vi "HAPS_PhaseGainSweep_Preamp_ICs.vi"() -> ()   [LabVIEW 2023, in "HAPS.lvlib"]
uses:
  HAPS.lvlib
  HAPS_SerialPort.ctl
  MCU_Function.ctl
  set_ele.ctl
  HAPS_MCU_ELE_Func.ctl
  R_S/R_S.lvlib
panel:
  out "Each_Phase_Sweep(sec)":dbl
  out "dup path":path
  out "Gain_step":i32
  out "channel":i32
  out "chain_id":i32
  out "group":i32
  out "array_id":i32
  in  "Gain_Start_Step":i32
  in  "Phase Sweep Step":i32=64
  in  "Gain Sweep Step":i32=36
  in  "comn_gain":i32=17
  in  "Init?":bool=TRUE
  in  "File_note":string
  out "Duration(sec)":dbl
  out "In-Phase : Phase(degree)":dbl[](graph)
  out "In-Phase : Gain(dB)":dbl[](graph)
  in  "Phase diff. Criteria":dbl format="%#_13g"
  in  "Tx/Rx":enum16{"Rx", "Tx"}(ring)=enum."Tx"
  in  "array_id (MCU index)":i32
  in  "MCU_UART_addr":refnum<visa-resource-name>="COM8"
  in  "Target(degree)":dbl format="%#_13g"
  in  "SweepPoints":i32=11
  in  "sParameter":i32=21
  in  "Stop_Freq(GHz)":dbl=39.5
  in  "Start_Freq(GHz)":dbl=38.5
  in  "VISA resource name":refnum<visa-resource-name>="TCPIP0::192.168.119.45::inst0::INSTR"
  in  "HAPS_Equipment":enum16{"Keysight", "R&S"}(ring)=enum."R&S"
  # "HAPS_24x24_PhaseGain_Sweep_Preamp_v1.4"
  # "K:4718\nR:2798"
  # "VNA"
  # "Test Status"
  # "DUT"
  # "TCPIP0::192.168.1.31::hislip0::INSTR"
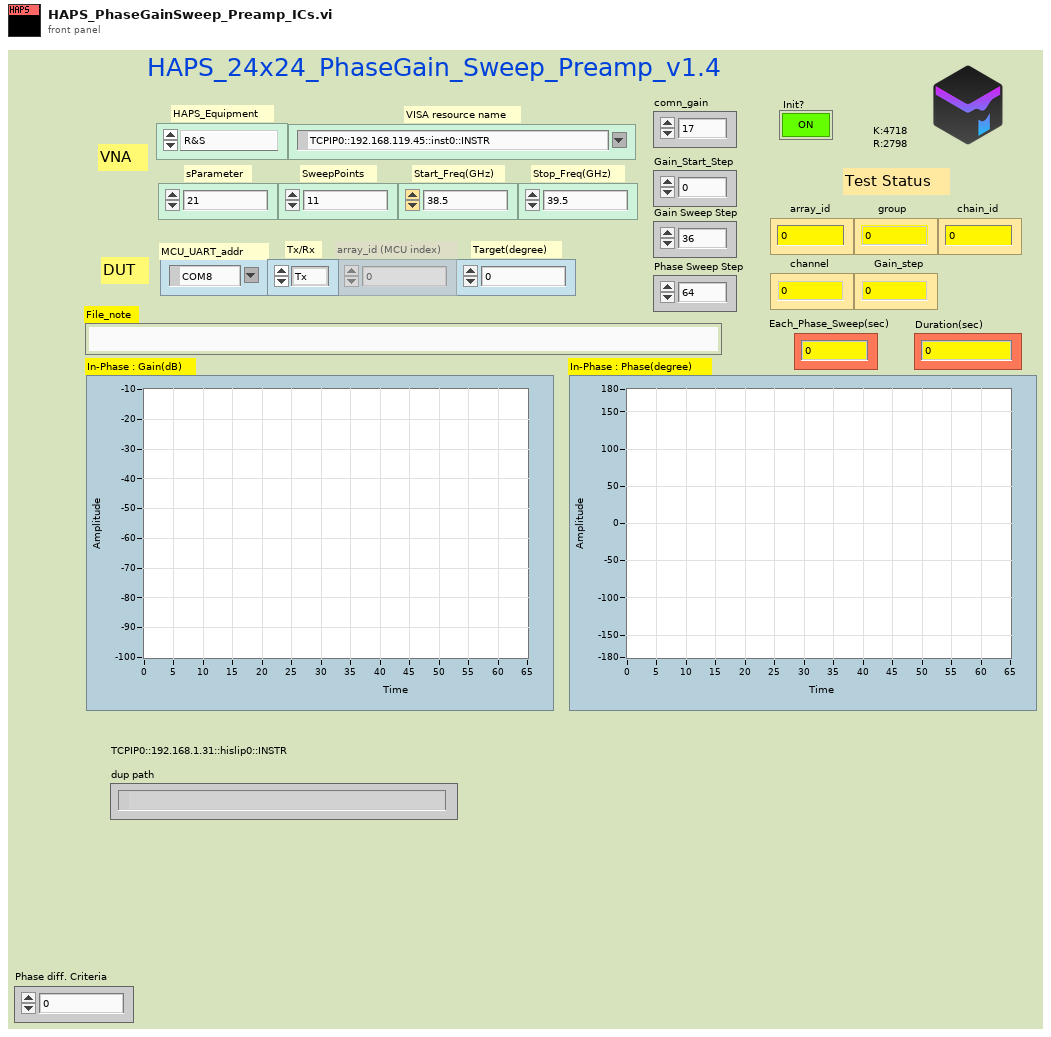
[diagram p1: front panel]
types:
  T1 = typedef "HAPS.lvlib/HAPS_SerialPort.ctl" = enum16{"Init", "Close", "CMD", "Flush"}
  T2 = typedef "HAPS.lvlib/HAPS_MCU_ELE_Func.ctl" = enum16{"array_init", "set_com_gain", "set_ch_gain_phase", "set_pd_range", "get_preamp_temp", "get_bfic_temp", "get_tx_pd", "ch_on", "ch_on_2", "ch_ctrl_all", "array_ctrl_src"}
  T3 = typedef "HAPS.lvlib/MCU_Function.ctl" = cluster{"Tx/Rx":enum16{"Rx", "Tx"}, "Enable?":enum16{"OFF", "On"}, "Source":enum16{"MCU", "ACU"}}
  T4 = typedef "HAPS.lvlib/set_ele.ctl" = cluster{"ch":i32, "chain_id":i32, "group":i32, "array_id":i32, "ele_phase":i32, "ele_gain":i32, "com_gain":i32, "pd_range":i32}
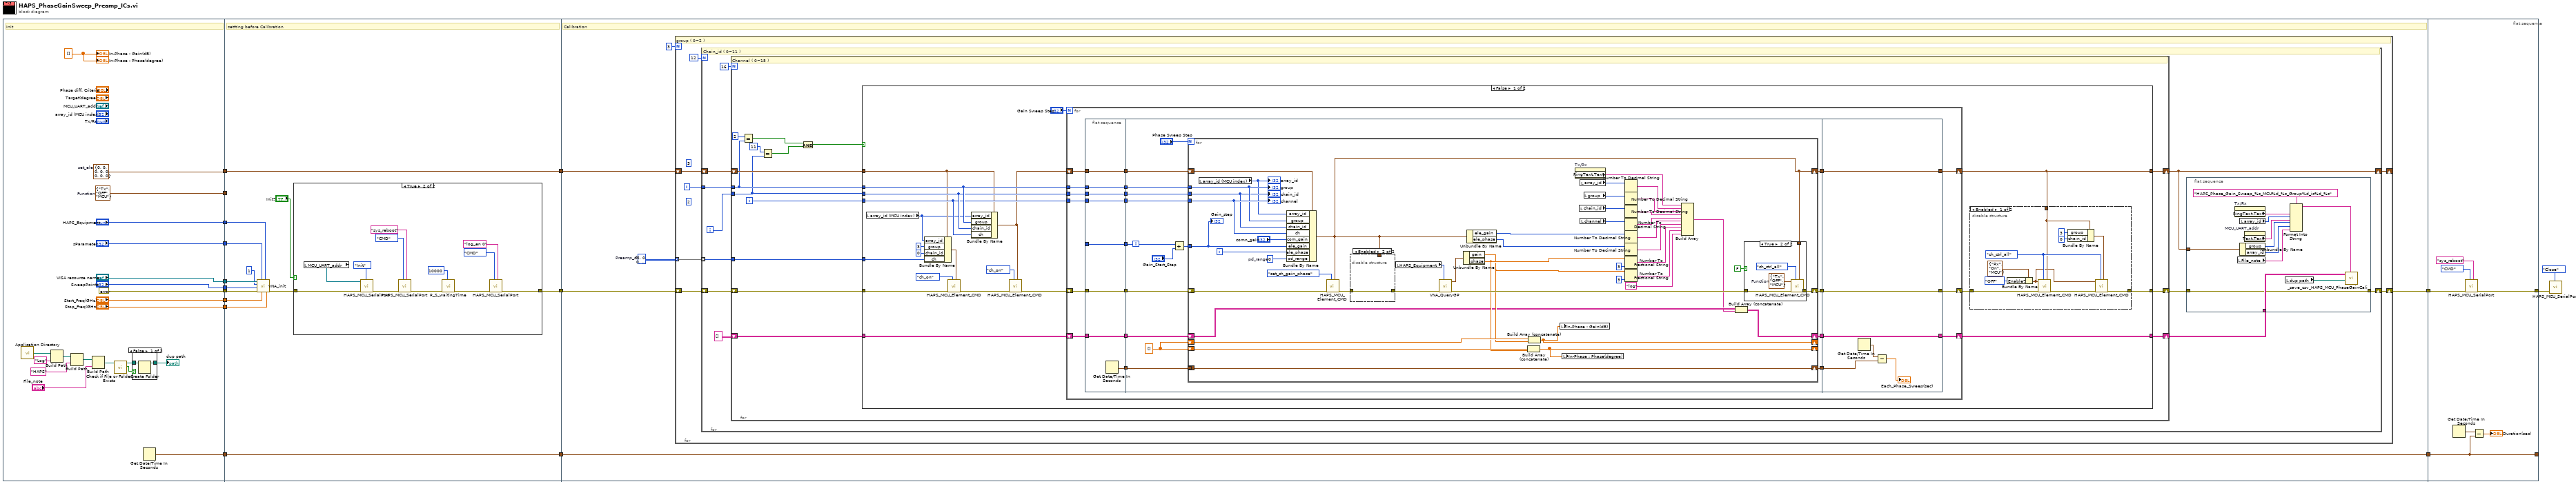
[diagram p0: block diagram]
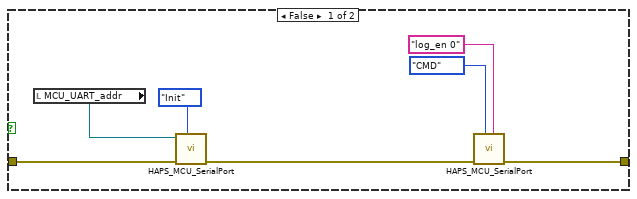
[diagram p3: hidden frame]
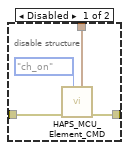
[diagram p4: hidden frame]
diagram:
  n1 = flat-sequence {
    tunnel: [w31] -> w17
    tunnel: [w38] -> w16
    tunnel: [errorcluster {"status"=FALSE, "code"=0, "source"=""} ("error in")] -> w14
    tunnel: ["sParameter"] -> w12
    tunnel: ["VISA resource name"] -> w11
    tunnel: ["Start_Freq(GHz)"] -> w10
    tunnel: ["Stop_Freq(GHz)"] -> w9
    tunnel: ["SweepPoints"] -> w8
    tunnel: ["HAPS_Equipment"] -> w7
    tunnel: [w28] -> w5
    tunnel: w17 -> [w54]
    tunnel: w16 -> [_]
    tunnel: [w54] -> w15
    tunnel: w14 -> [w53]
    tunnel: [w45] -> w13
    tunnel: w12 -> [w52]
    tunnel: w11 -> [w51]
    tunnel: w10 -> [w50]
    tunnel: w9 -> [w49]
    tunnel: w8 -> [w48]
    tunnel: w7 -> [w44]
    tunnel: [w43] -> w6
    tunnel: w5 -> [w43]
    tunnel: w15 -> [w78]
    tunnel: w13 -> [w79]
    tunnel: w6 -> [w76]
    tunnel: [w76] -> w4
    tunnel: [w74] -> w3
    tunnel: [w276] -> _
    tunnel: w4 -> [w276]
    tunnel: w3 -> [w272]
    tunnel: [w271] -> w2
    frame #0 {
      w29 = dbl[] []
      w31 = T4 {"ch"=0, "chain_id"=0, "group"=0, "array_id"=0, "ele_phase"=0, "ele_gain"=0, "com_gain"=0, "pd_range"=0}  # set_ele
      w38 = T3 {"Tx/Rx"=enum."Tx", "Enable?"=enum."OFF", "Source"=enum."MCU"}  # Function
      # "Init"
      n2 = call <vilib>:"Application Directory.vi"() -> ("Application Directory"=w26:path)
      n3 = Build Path(base path=w26, name or relative path="Log") -> (appended path=w27:path)
      n4 = Build Path(base path=w27, name or relative path="HAPS") -> (appended path=w23:path)
      n5 = Build Path(base path=w23, name or relative path="File_note") -> (appended path=w21:path)
      n6 = call <vilib>:"Check if File or Folder Exists.vi"("path"=w21) -> ("file or folder exists?"=w20:bool, "dup path"=w19:path)  [unwired: 8 in, 1 out]
      n7 = case shown="False" w20 {
        tunnel: w19 -> [w40 w41]
        tunnel: [w39 w41] -> w18
        frame False {
          n8 = Create Folder(path (use dialog)=w40) -> (created path=w39:path)  [unwired: 2 in, 2 out]
        }
        frame True {
        }
      }
      "dup path" <- w18
      n9 = Get Date/Time In Seconds() -> (seconds since 1Jan1904=w28:timestamp)
      "In-Phase : Gain(dB)" <- w29
      "In-Phase : Phase(degree)" <- w29
    }
    frame #1 {
      # "settting before Calibration"
      n10 = call "VNA_init.vi"("Stop_Freq(GHz)"=w49, "HAPS_MCU_CMD"=w44, "Start_Freq(GHz)"=w50, "sParameter"=w52, "error in"=w53, "SweepPoints"=w48, "Mark no."=1, "VISA resource name"=w51) -> ("error out"=w46:errorcluster)  [unwired: 3 in]
      n11 = case shown="True" "Init?" {
        tunnel: w46 -> [w58 w71]
        tunnel: [w55 w68] -> w45
        frame False {
          n12 = local read "MCU_UART_addr"() -> (w56:refnum<visa-resource-name>)
          n13 = call "HAPS_MCU_SerialPort.vi"("HAPS_SerialPort_Func"=HAPS_SerialPort."Init", "error in"=w58, "VISA resource name"=w56) -> ("error out"=w59:errorcluster)  [unwired: 6 in, 2 out]
          n14 = call "HAPS_MCU_SerialPort.vi"("Command"="log_en 0", "HAPS_SerialPort_Func"=enum16{"Init", "Close", "CMD"}."CMD" ("HAPS_SerialPort"), "error in"=w59) -> ("error out"=w55:errorcluster)  [unwired: 6 in, 2 out]
        }
        frame True {
          n15 = local read "MCU_UART_addr"() -> (w69:refnum<visa-resource-name>)
          n16 = call "HAPS_MCU_SerialPort.vi"("HAPS_SerialPort_Func"=HAPS_SerialPort."Init", "error in"=w71, "VISA resource name"=w69) -> ("error out"=w65:errorcluster)  [unwired: 6 in, 2 out]
          n17 = call "HAPS_MCU_SerialPort.vi"("Command"="sys_reboot", "HAPS_SerialPort_Func"=enum16{"Init", "Close", "CMD"}."CMD" ("HAPS_SerialPort"), "error in"=w65) -> ("error out"=w64:errorcluster)  [unwired: 6 in, 2 out]
          n18 = call "R_S_waitingTime.vi"("Waiting Time(ms)"=u32 10000, "error in"=w64) -> ("error out"=w63:errorcluster)  [unwired: 9 in]
          n19 = call "HAPS_MCU_SerialPort.vi"("Command"="log_en 0", "HAPS_SerialPort_Func"=enum16{"Init", "Close", "CMD"}."CMD" ("HAPS_SerialPort"), "error in"=w63) -> ("error out"=w68:errorcluster)  [unwired: 6 in, 2 out]
        }
      }
    }
    frame #2 {
      w75 = i32[][] [[2, 0, 0, 8, 8, 10, 11, 9, 9, 1, 1, 3], [3, 1, 1, 9, 9, 11, 13, 15, 15, 7, 7, 5], [5, 7, 7, 15, 15, 13, 14, 14, 6, 6, 4, 12]]  # Preamp_ch
      # "Calibration"
      n20 = for {
        N: 3 -> [_]
        shift-right: [w80] -> _
        shift-left: w78 -> [w84]
        shift-right: [w86] -> w74
        shift-left: w79 -> [w85]
        tunnel: w75 -> [w81] mode=indexing
        i -> [w82]
        (unwired) 2
        (unwired) 3
        # "group ( 0~2 )"
        n21 = for {
          N: 12 -> [_]
          shift-right: [w91] -> w80
          shift-left: w84 -> [w95]
          shift-right: [w87] -> w86
          shift-left: w85 -> [w96]
          tunnel: w82 -> [w94]
          tunnel: w81 -> [w92] mode=indexing
          i -> [w93]
          # "Chain_id ( 0~11 )"
          n22 = for {
            N: 16 -> [_]
            shift-right: [w121] -> w91
            shift-left: w95 -> [w124]
            shift-right: [w119] -> w90
            shift-left: string[][] [] -> [w120]
            shift-right: [w122] -> w88
            shift-left: w96 -> [w123]
            tunnel: w94 -> [w118]
            tunnel: w93 -> [w111]
            tunnel: w92 -> [w110]
            i -> [w112]
            # "Channel ( 0~15 )"
            n23 = Equal?(x=2, y=w118) -> (x = y?=w115:bool)
            n24 = Equal?(x=11, y=w111) -> (x = y?=w114:bool)
            n25 = And(x=w115, y=w114) -> (x .and. y?=w113:bool)
            n26 = case shown="False" w113 {
              tunnel: w124 -> [w133 w269]
              tunnel: w112 -> [w142 _]
              tunnel: w123 -> [w134 w268]
              tunnel: w118 -> [w144 _]
              tunnel: w111 -> [w143 _]
              tunnel: [w138 w268] -> w122
              tunnel: [w137 w269] -> w121
              tunnel: w120 -> [w145 w270]
              tunnel: [w126 w270] -> w119
              tunnel: w110 -> [w128 _]
              frame False {
                n27 = local read "array_id (MCU index)"() -> (w131:i32)
                n28 = Bundle By Name(cluster=w133, "array_id"=w131, "group"=3, "chain_id"=0, "ch"=w128) -> (w132:T4)
                n29 = call "HAPS_MCU_Element_CMD.vi"("set_ele"=w132, "HAPS_MCU_ELE_Func."=HAPS_MCU_ELE_Func."ch_on", "error in"=w134) -> ("error out"=w135:errorcluster)  [unwired: 7 in, 1 out]
                n30 = Bundle By Name(cluster=w133, "array_id"=w131, "group"=w144, "chain_id"=w143, "ch"=w142) -> (w127:T4)
                n31 = call "HAPS_MCU_Element_CMD.vi"("set_ele"=w127, "HAPS_MCU_ELE_Func."=HAPS_MCU_ELE_Func."ch_on", "error in"=w135) -> ("error out"=w140:errorcluster)  [unwired: 7 in, 1 out]
                n32 = for {
                  N: "Gain Sweep Step" -> [_]
                  tunnel: w144 -> [w166]
                  tunnel: w143 -> [w165]
                  tunnel: w142 -> [w164]
                  shift-right: [w162] -> w139
                  shift-left: w140 -> [w163]
                  shift-right: [w161] -> w137
                  shift-left: w127 -> [w160]
                  shift-right: [w159] -> w126
                  shift-left: w145 -> [w167]
                  i -> [w158]
                  n33 = flat-sequence {
                    tunnel: w158 -> [w169]
                    tunnel: w160 -> [w170]
                    tunnel: w163 -> [w171]
                    tunnel: w164 -> [w172]
                    tunnel: w165 -> [w173]
                    tunnel: w166 -> [w174]
                    tunnel: w167 -> [w175]
                    tunnel: [w175] -> w157
                    tunnel: [w174] -> w156
                    tunnel: [w173] -> w155
                    tunnel: [w172] -> w154
                    tunnel: [w171] -> w153
                    tunnel: [w170] -> w152
                    tunnel: [w169] -> w151
                    tunnel: [w168] -> w150
                    tunnel: w157 -> [w190]
                    tunnel: w156 -> [w189]
                    tunnel: w155 -> [w188]
                    tunnel: w154 -> [w187]
                    tunnel: w153 -> [w186]
                    tunnel: w152 -> [w183]
                    tunnel: w151 -> [w181]
                    tunnel: w150 -> [w177]
                    tunnel: [w185] -> w149
                    tunnel: [w184] -> w148
                    tunnel: [w182] -> w147
                    tunnel: [w176] -> w146
                    tunnel: [w253] -> w159
                    tunnel: [w254] -> w161
                    tunnel: [w255] -> w162
                    tunnel: w149 -> [w255]
                    tunnel: w148 -> [w254]
                    tunnel: w147 -> [w253]
                    tunnel: w146 -> [w250]
                    frame #0 {
                      n34 = Get Date/Time In Seconds() -> (seconds since 1Jan1904=w168:timestamp)
                    }
                    frame #1 {
                      w178 = dbl[] []
                      n35 = Add(x=w181, y="Gain_Start_Step") -> (x+y=w180:i32)
                      n36 = for {
                        N: "Phase Sweep Step" -> [_]
                        tunnel: w187 -> [w237]
                        tunnel: w189 -> [w235]
                        tunnel: w188 -> [w234]
                        shift-right: [w215] -> _
                        shift-left: w178 -> [w217]
                        shift-right: [w214] -> _
                        shift-left: w178 -> [w216]
                        shift-right: [w212] -> w185
                        shift-left: w186 -> [w236]
                        shift-right: [w202] -> w184
                        shift-left: w183 -> [w238]
                        shift-right: [w206] -> w182
                        shift-left: w190 -> [w208]
                        tunnel: w180 -> [w194]
                        tunnel: w177 -> [w193]
                        shift-right: [w193] -> w176
                        shift-left: _ -> [_]
                        i -> [w192]
                        w232 = 0  # pd_range
                        n37 = local read "array_id (MCU index)"() -> (w230:i32)
                        "array_id" <- w230
                        n38 = Bundle By Name(cluster=w238, "array_id"=w230, "group"=w235, "chain_id"=w234, "ch"=w237, "com_gain"="comn_gain", "ele_gain"=w194, "ele_phase"=w192, "pd_range"=w232) -> (w202:T4)
                        n39 = call "HAPS_MCU_Element_CMD.vi"("set_ele"=w202, "HAPS_MCU_ELE_Func."=HAPS_MCU_ELE_Func."set_ch_gain_phase", "error in"=w236) -> ("error out"=w204:errorcluster)  [unwired: 7 in, 1 out]
                        n40 = disable-structure shown="Enabled" {
                          disable-tunnel: w204 -> [w242 w243]
                          disable-tunnel: [w241 w243] -> w203
                          disable-tunnel: w202 -> [w239 _]
                          frame Disabled {
                            n41 = call "HAPS_MCU_Element_CMD.vi"("set_ele"=w239, "HAPS_MCU_ELE_Func."=HAPS_MCU_ELE_Func."ch_on", "error in"=w242) -> ("error out"=w241:errorcluster)  [unwired: 7 in, 1 out]
                          }
                          frame Enabled {
                          }
                        }
                        n42 = local read "HAPS_Equipment"() -> (w219:enum16{"Keysight", "R&S"})
                        n43 = call "VNA_QueryGP.vi"("HAPS_Equipment"=w219, "error in"=w203) -> ("error out"=w213:errorcluster, "queryMarker"=w218:cluster{"gain":dbl, "phase":dbl})  [unwired: 8 in]
                        n44 = Unbundle By Name(w218) -> ("gain"=w209:dbl, "phase"=w210:dbl)
                        n45 = Unbundle By Name(w202) -> ("ele_gain"=w195:i32, "ele_phase"=w211:i32)
                        n46 = Build Array (concatenate)(w216, w210) -> (w214:dbl[])
                        n47 = Build Array (concatenate)(w217, w209) -> (w215:dbl[])
                        n48 = local write "In-Phase : Gain(dB)"(w215) -> ()
                        n49 = local write "In-Phase : Phase(degree)"(w214) -> ()
                        n50 = property on="Tx/Rx" class="Enum (strict)"() -> ("RingText.Text"=w196:string)  [unwired: 2 in, 2 out]
                        n51 = local read "chain_id"() -> (w221:i32)
                        n52 = local read "array_id"() -> (w223:i32)
                        n53 = local read "channel"() -> (w220:i32)
                        n54 = local read "group"() -> (w222:i32)
                        n55 = Number To Decimal String(number=w223) -> (decimal integer string=w197:string)  [unwired: 1 in]
                        n56 = Number To Decimal String(number=w222) -> (decimal integer string=w198:string)  [unwired: 1 in]
                        n57 = Number To Decimal String(number=w221) -> (decimal integer string=w199:string)  [unwired: 1 in]
                        n58 = Number To Decimal String(number=w220) -> (decimal integer string=w200:string)  [unwired: 1 in]
                        n59 = Number To Decimal String(number=w195) -> (decimal integer string=w201:string)  [unwired: 1 in]
                        n60 = Number To Decimal String(number=w211) -> (decimal integer string=w224:string)  [unwired: 1 in]
                        n61 = Number To Fractional String(number=w210, precision (6)=i16 3) -> (F-format string=w227:string)  [unwired: 2 in]
                        n62 = Number To Fractional String(number=w209, precision (6)=i16 3) -> (F-format string=w228:string)  [unwired: 2 in]
                        n63 = Build Array(w196, w197, w198, w199, w200, w201, w224, w227, w228, "log") -> (w207:string[])
                        n64 = Build Array (concatenate)(w208, w207) -> (w206:string[][])
                        n65 = case shown="True" FALSE {
                          tunnel: w213 -> [w244 w247]
                          tunnel: [w244 w246] -> w212
                          tunnel: w202 -> [_ w245]
                          frame False {
                          }
                          frame True {
                            w249 = T3 {"Tx/Rx"=enum."Tx", "Enable?"=enum."OFF", "Source"=enum."MCU"}  # Function
                            n66 = call "HAPS_MCU_Element_CMD.vi"("set_ele"=w245, "HAPS_MCU_ELE_Func."=HAPS_MCU_ELE_Func."ch_ctrl_all", "error in"=w247, "Function"=w249) -> ("error out"=w246:errorcluster)  [unwired: 6 in, 1 out]
                          }
                        }
                        "group" <- w235
                        "chain_id" <- w234
                        "channel" <- w237
                        "Gain_step" <- w194
                      }
                    }
                    frame #2 {
                      n67 = Get Date/Time In Seconds() -> (seconds since 1Jan1904=w251:timestamp)
                      n68 = Subtract(x=w251, y=w250) -> (x-y=→"Each_Phase_Sweep(sec)":dbl)
                    }
                  }
                }
                n69 = disable-structure shown="Enabled" {
                  disable-tunnel: w139 -> [w266 w267]
                  disable-tunnel: [w262 w267] -> w138
                  disable-tunnel: w137 -> [w257 _]
                  frame Enabled {
                    w261 = HAPS_MCU_ELE_Func."ch_ctrl_all" ("HAPS_MCU_ELE_Func.")
                    n70 = Bundle By Name(cluster=T3 {"Tx/Rx"=enum."Rx", "Enable?"=enum."On", "Source"=enum."MCU"} ("Function"), "Enable?"=enum16{"OFF", "On"}."OFF") -> (w260:T3)
                    n71 = call "HAPS_MCU_Element_CMD.vi"("set_ele"=w257, "HAPS_MCU_ELE_Func."=w261, "error in"=w266, "Function"=w260) -> ("error out"=w263:errorcluster)  [unwired: 6 in, 1 out]
                    n72 = Bundle By Name(cluster=w257, "group"=3, "chain_id"=0) -> (w256:T4)
                    n73 = call "HAPS_MCU_Element_CMD.vi"("set_ele"=w256, "HAPS_MCU_ELE_Func."=w261, "error in"=w263, "Function"=w260) -> ("error out"=w262:errorcluster)  [unwired: 6 in, 1 out]
                  }
                  frame Disabled {
                  }
                }
              }
              frame True {
              }
            }
          }
          n74 = flat-sequence {
            tunnel: w91 -> [w103]
            tunnel: w90 -> [w100]
            tunnel: w88 -> [w98]
            tunnel: [w98] -> w87
            frame #0 {
              n75 = property on="Tx/Rx" class="Enum (strict)"() -> ("RingText.Text"=w107:string)  [unwired: 2 in, 2 out]
              n76 = local read "File_note"() -> (w101:string)
              n77 = local read "array_id"() -> (w106:i32)
              n78 = Unbundle By Name(w103) -> ("group"=w105:i32, "array_id"=w102:i32)
              n79 = property on="MCU_UART_addr" class="VISAName"() -> ("Text.Text"=w109:string)  [unwired: 2 in, 2 out]
              n80 = local read "dup path"() -> (w99:path)
              n81 = Format Into String(format string="HAPS_Phase_Gain_Sweep_%s_MCU%d_%s_Group%d_ic%d_%s", w107, w106, w109, w105, w102, w101) -> (resulting string=w108:string)  [unwired: 2 in, 1 out]
              n82 = call "_save_csv_HAPS_MCU_PhaseGainCali.vi"("NoteName"=w108, "dup path"=w99, "array in"=w100) -> ()  [unwired: 8 in, 1 out]
            }
          }
        }
      }
    }
    frame #3 {
      n83 = Get Date/Time In Seconds() -> (seconds since 1Jan1904=w277:timestamp)
      n84 = call "HAPS_MCU_SerialPort.vi"("Command"="sys_reboot", "HAPS_SerialPort_Func"=enum16{"Init", "Close", "CMD"}."CMD" ("HAPS_SerialPort"), "error in"=w272) -> ("error out"=w271:errorcluster)  [unwired: 6 in, 2 out]
      n85 = Subtract(x=w277, y=w276) -> (x-y=→"Duration(sec)":dbl)
    }
  }
  n86 = call "HAPS_MCU_SerialPort.vi"("HAPS_SerialPort_Func"=HAPS_SerialPort."Close", "error in"=w2) -> ()  [unwired: 7 in, 3 out]
